vi "Helper - Export - Sine.vi"() -> (3 "Sine with Noise":dbl[](array[numeric]))   [LabVIEW 2023]
doc: "Generates a Sine signal with noise."
panel:
  # "Generates a Sine signal with noise."
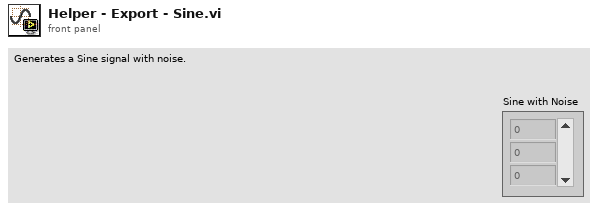
[diagram p1: front panel]
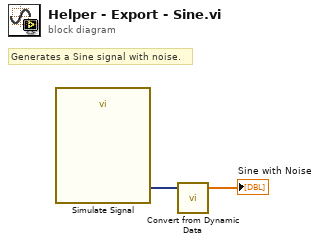
[diagram p0: block diagram]
diagram:
  # "Generates a Sine signal with noise."
  n1 = call "Simulate Signal"() -> ("Sine with Uniform Noise"=w2:dynamicdata)  [unwired: 14 in, 1 out]
  n2 = call "Convert from Dynamic Data"("Dynamic Data Type"=w2) -> ("Array"=→"Sine with Noise":dbl[])  [unwired: 3 in]
